vi "SIM Newton-Raphson step.vi"(10 "Factored Jacobian":T1, 11 "F(y_current)":dbl[](array[numeric])) -> (0 "Newton Error?":bool, 3 "y next minus y current":dbl[](array[numeric]))   [LabVIEW 2010]
uses:
  SIM Factored Matrix.ctl
  lvanlys.dll
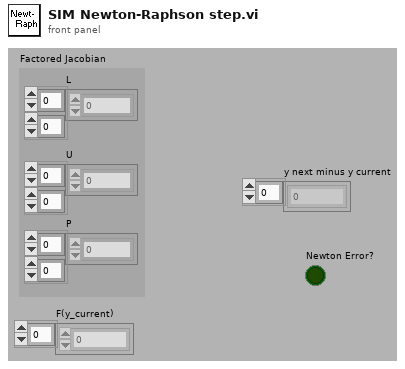
[diagram p1: front panel]
types:
  T1 = typedef "SIM Factored Matrix.ctl" = cluster{"L":dbl[][], "U":dbl[][], "P":i32[][]}
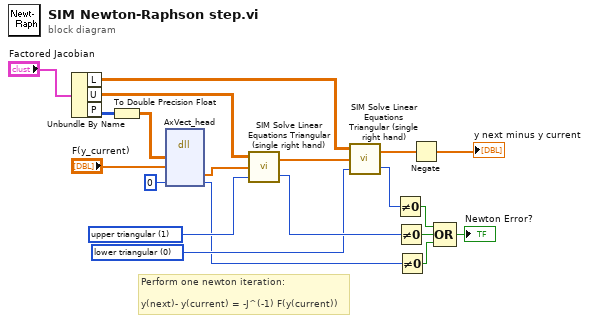
[diagram p0: block diagram]
diagram:
  w7 = 0 items=["lower triangular", "upper triangular", "symmetric matrix"] ("matrix type")
  w8 = 1 items=["lower triangular", "upper triangular", "symmetric matrix"] ("matrix type")
  # "Perform one newton iteration:\n\ny(next)- y(current) = -J^(-1) F(y(current))"
  n1 = Unbundle By Name("Factored Jacobian") -> ("L"=w16:dbl[][], "U"=w15:dbl[][], "P"=w2:i32[][])
  n2 = To Double Precision Float(number=w2) -> (double precision float=w1:dbl[][])
  n3 = dll-call lib="C:/Program Files/National Instruments/LabVIEW 2010/resource/lvanlys.*" fn="AxVect_head" label="A x Vector"("aHandle"=w1, "xHandle"="F(y_current)", "dsperr"=0 ("output param")) -> ("Known Vector"=w4:dbl[], "dsperr"=w3:i32)  [unwired: 5 in, 4 out]
  n4 = call "SIM Solve Linear Equations Triangular (single right hand).vi"("matrix type"=w8, "Known Vector"=w4, "Input Matrix"=w15) -> ("error"=w10:i32, "Solution Vector"=w20:dbl[])
  n5 = call "SIM Solve Linear Equations Triangular (single right hand).vi"("matrix type"=w7, "Known Vector"=w20, "Input Matrix"=w16) -> ("error"=w13:i32, "Solution Vector"=w19:dbl[])
  n6 = Not Equal To 0?(x=w13) -> (x != 0?=w14:bool)
  n7 = Not Equal To 0?(x=w10) -> (x != 0?=w12:bool)
  n8 = Not Equal To 0?(x=w3) -> (x != 0?=w11:bool)
  n9 = Negate(x=w19) -> (-x=→"y next minus y current":dbl[])
  n10 = Compound Arithmetic op=OR(w14, w12, w11) -> (→"Newton Error?":bool)
